vi "mouse_parse_packet.vi"(0 "Data in":string) -> (3 "Full packet?":bool, 4 "Delta x":i16, 5 "Delta y":i16)   [LabVIEW 2012]
panel:
  out "Heading":i16
  # "Heading not used"
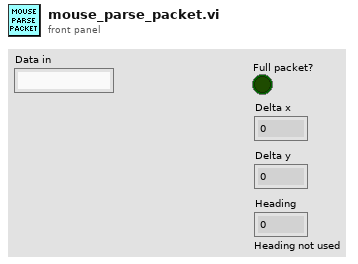
[diagram p1: front panel]
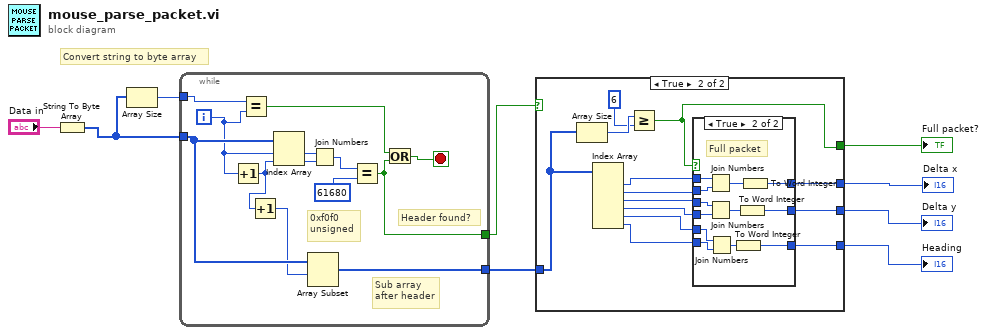
[diagram p0: block diagram]
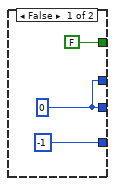
[diagram p2: hidden frame]
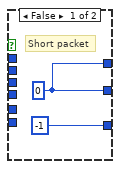
[diagram p3: hidden frame]
diagram:
  # "Convert string to byte array"
  n1 = String To Byte Array(string="Data in") -> (unsigned byte array=w8:u8[])
  n2 = Array Size(array=w8) -> (size(s)=w7:i32)
  n3 = while {
    tunnel: w8 -> [w17]
    tunnel: [w16] -> w5
    tunnel: w7 -> [w15]
    tunnel: [w11] -> w6
    i -> [w14]
    stop <- w12 stop-if-true
    # "Header found?"
    # "Sub array \nafter header"
    # "0xf0f0\nunsigned"
    n4 = Increment(x=w14) -> (x+1=w18:i32)
    n5 = Equal?(x=w15, y=w14) -> (x = y?=w13:bool)
    n6 = Increment(x=w18) -> (x+1=w10:i32)
    n7 = Index Array(array=w17, index #1=w14, index #2=w18) -> (element #1=w21:u8, element #2=w22:u8)
    n8 = Array Subset(array=w17, index=w10) -> (w16:u8[])  [unwired: 1 in]
    n9 = Join Numbers(hi=w21, lo=w22) -> ((hi.lo)=w20:u16)
    n10 = Equal?(x=w20, y=u16 61680) -> (x = y?=w11:bool)
    n11 = Or(x=w13, y=w11) -> (x .or. y?=w12:bool)
  }
  n12 = case shown="True" w6 {
    tunnel: w5 -> [_ w32]
    tunnel: [w25 w31] -> w3
    tunnel: [w25 w30] -> w2
    tunnel: [i16 -1 w29] -> w1
    tunnel: [FALSE w28] -> w4
    frame False {
      w25 = i16 0
    }
    frame True {
      n13 = Array Size(array=w32) -> (size(s)=w27:i32)
      n14 = Index Array(array=w32) -> (element #1=w38:u8, element #2=w37:u8, element #3=w36:u8, element #4=w35:u8, element #5=w34:u8, element #6=w33:u8)  [unwired: 6 in]
      n15 = Greater Or Equal?(x=w27, y=6 ("x")) -> (x >= y?=w28:bool)
      n16 = case shown="True" w28 {
        tunnel: w38 -> [_ w52]
        tunnel: w37 -> [_ w51]
        tunnel: w36 -> [_ w50]
        tunnel: w35 -> [_ w49]
        tunnel: [w40 w42] -> w31
        tunnel: [w40 w41] -> w30
        tunnel: w34 -> [_ w46]
        tunnel: w33 -> [_ w45]
        tunnel: [i16 -1 w43] -> w29
        frame False {
          w40 = i16 0
          # "Short packet"
        }
        frame True {
          # "Full packet"
          n17 = Join Numbers(hi=w52, lo=w51) -> ((hi.lo)=w48:u16)
          n18 = Join Numbers(hi=w50, lo=w49) -> ((hi.lo)=w47:u16)
          n19 = Join Numbers(hi=w46, lo=w45) -> ((hi.lo)=w44:u16)
          n20 = To Word Integer(number=w44) -> (16bit integer=w43:i16)
          n21 = To Word Integer(number=w47) -> (16bit integer=w41:i16)
          n22 = To Word Integer(number=w48) -> (16bit integer=w42:i16)
        }
      }
    }
  }
  "Full packet?" <- w4
  "Delta x" <- w3
  "Delta y" <- w2
  "Heading" <- w1
